vi "Acquire average image (SubVI).vi"(9 "Camera type":T4(ring), 10 "Measurement camera cluster in":T3, 11 "averaging time (ms)":u32=1000) -> (3 "Refnum out":T2)   [LabVIEW 2012]
uses:
  <vilib>/vision/Image Controls.llb/IMAQ Image.ctl
  <vilib>/userdefined/High Color/IMAQdx.ctl
  Global variables.vi
  <vilib>/vision/driver/imaqhl.llb/IMAQ Grab Acquire.vi
  <vilib>/vision/driver/IMAQdx.llb/IMAQdx Grab.vi
  <vilib>/vision/driver/imaqll.llb/IMAQ Extract Buffer.vi
  <vilib>/vision/NI_Vision_Development_Module.lvlib
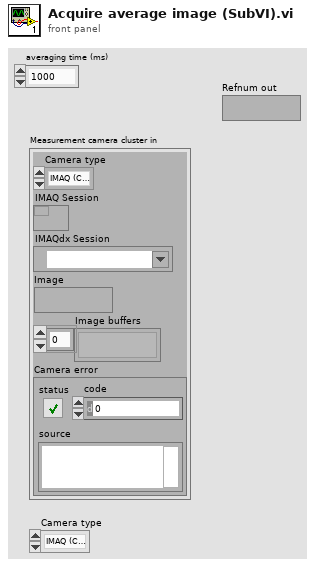
[diagram p1: front panel]
types:
  T1 = typedef "IMAQdx.ctl" = refnum<k21>
  T2 = typedef "IMAQ Image.ctl" = refnum<image>
  T3 = cluster{"Camera type":enum16{"IMAQ (Camera Link)", "IMAQ ring", "IMAQdx (firewire)", "No camera"}, "IMAQ Session":refnum<k11>, "IMAQdx Session":T1, "Image":T2, "Image buffers":T2[], "Camera error":errorcluster}
  T4 = enum16{"IMAQ (Camera Link)", "IMAQ ring", "IMAQdx (firewire)", "No camera"}
  T5 = typedef "Image Type" = u32
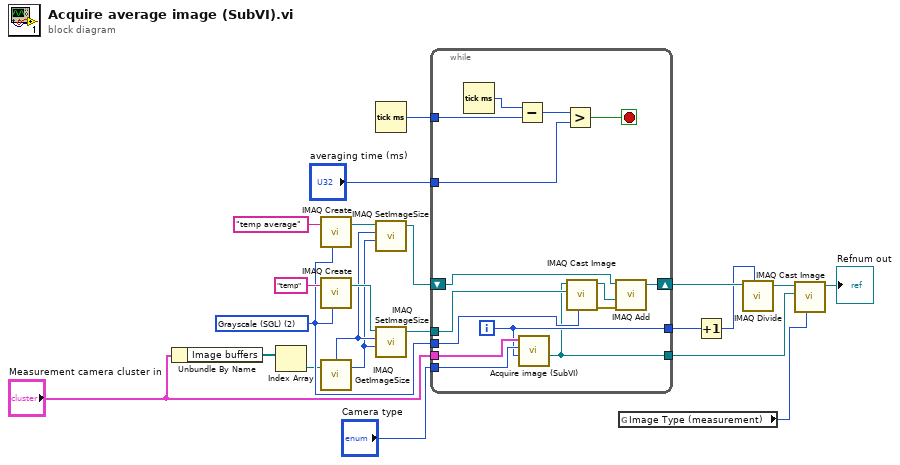
[diagram p0: block diagram]
diagram:
  w19 = T5 2 items=["Grayscale (U8)", "Grayscale (I16)", "Grayscale (SGL)", "Complex (CSG)", "RGB (U32)", "HSL (U32)", "RGB (U64)", "Grayscale (U16)"] ("Image Type")
  n1 = Unbundle By Name("Measurement camera cluster in") -> ("Image buffers"=w8:T2[])
  n2 = Index Array(array=w8) -> (element=w7:T2)  [unwired: 1 in]
  n3 = call "IMAQ Create"("Image Name"="temp average", "Image Type"=w19) -> ("New Image"=w6:T2)  [unwired: 3 in, 1 out]
  n4 = call "IMAQ Create"("Image Name"="temp", "Image Type"=w19) -> ("New Image"=w4:T2)  [unwired: 3 in, 1 out]
  n5 = call "IMAQ GetImageSize"("Image"=w7) -> ("Y Resolution"=w1:i32, "X Resolution"=w2:i32)  [unwired: 3 in, 1 out]
  n6 = Tick Count (ms)() -> (millisecond timer value=w11:u32)
  n7 = call "IMAQ SetImageSize"("Y Resolution"=w1, "X Resolution"=w2, "Image"=w6) -> ("Image Out"=w5:T2)  [unwired: 2 in, 1 out]
  n8 = call "IMAQ SetImageSize"("Y Resolution"=w1, "X Resolution"=w2, "Image"=w4) -> ("Image Out"=w3:T2)  [unwired: 2 in, 1 out]
  n9 = while {
    tunnel: "Measurement camera cluster in" -> [w37]
    tunnel: "Camera type" -> [w36]
    tunnel: w19 -> [w35]
    tunnel: w3 -> [w34]
    shift-right: [w32] -> w18
    shift-left: w5 -> [w24]
    tunnel: [w31] -> w17
    tunnel: [w30] -> w14
    tunnel: w11 -> [w28]
    tunnel: "averaging time (ms)" -> [w25]
    i -> [w31]
    stop <- w26 stop-if-true
    n10 = Tick Count (ms)() -> (millisecond timer value=w29:u32)
    n11 = Subtract(x=w29, y=w28) -> (x-y=w27:u32)
    n12 = call "Acquire image (SubVI).vi"("Buffer number"=w31, "Camera type"=w36, "Measurement camera \ncluster in"=w37) -> ("Image Out"=w30:T2)  [unwired: 6 in, 2 out]
    n13 = Greater?(x=w27, y=w25) -> (0:w26:bool)
    n14 = call "IMAQ Cast Image"("Image Type"=w35, "Image Dst"=w34, "Image Src"=w30) -> ("error out"=w33:errorcluster, "Image Dst Out"=w23:T2)  [unwired: 7 in]
    n15 = call "IMAQ Add"("Image Src A"=w24, "Image Src B"=w23, "error in (no error)"=w33) -> ("Image Dst Out"=w32:T2)  [unwired: 4 in, 1 out]
  }
  n16 = global read "Global variables.vi" "Image Type (measurement)"() -> (w12:T5)
  n17 = Increment(x=w17) -> (x+1=w16:i32)
  n18 = call "IMAQ Divide"("Image Src A"=w18, "Constant"=w16) -> ("Image Dst Out"=w15:T2)  [unwired: 5 in, 1 out]
  n19 = call "IMAQ Cast Image"("Image Type"=w12, "Image Dst"=w14, "Image Src"=w15) -> ("Image Dst Out"=→"Refnum out":T2)  [unwired: 7 in, 1 out]
